vi "Page_Advanced_ReadAll.vi"(6 "ctl references":T1, 8 "error in (no error)":errorcluster, 10 "Calculated IncludeHWConfig":bool, 11 "AB_DLL in":refnum<class "AB_DLL.lvclass">) -> (0 "error out":errorcluster, 3 "AB_DLL out":refnum<class "AB_DLL.lvclass">)   [LabVIEW 2020, in "AB_DLL.lvclass"]
uses:
  <vilib>/AppBuilder/AB_Classes/DLL/AB_DLL.lvclass
  e:/builds/penguin/labview/branches/2020/dev/dist/vi.lib/AppBuilder/AB_Classes/TargetFile/AB_Targetfile.lvclass
  <resource>/Framework/Providers/Builds/AppBuilder/AB_UI_Page_Advanced_References.ctl
  <vilib>/AppBuilder/AB_Classes/DLL/AB_DLL.lvclass/AB_DLL.ctl
  <vilib>/AppBuilder/AB_Classes/Application/AB_Application.lvclass
  <vilib>/AppBuilder/AB_Classes/TargetFile/AB_Targetfile.lvclass
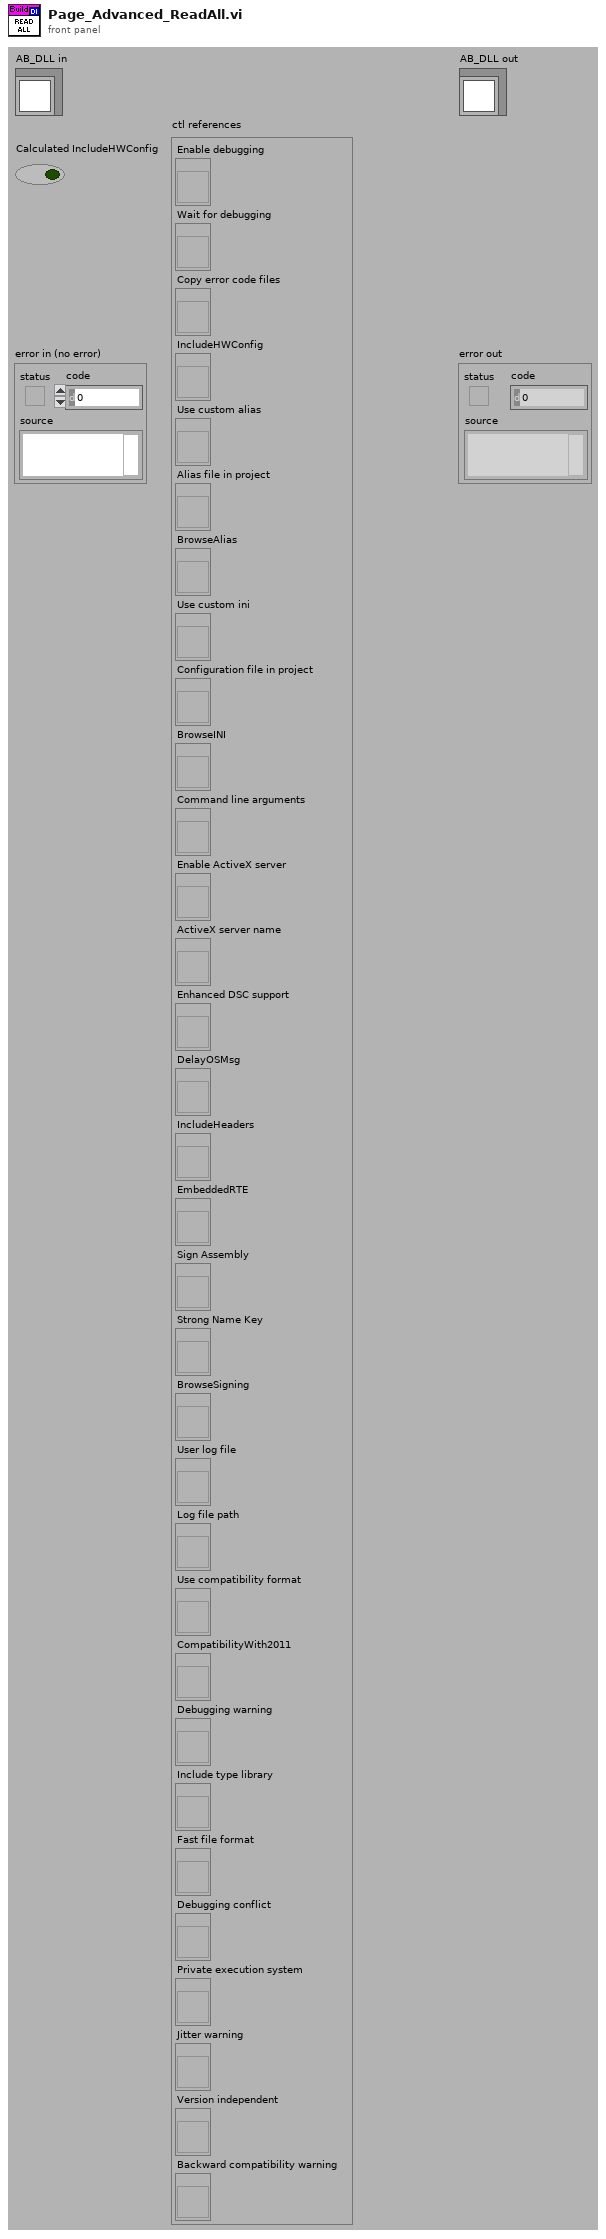
[diagram p1: front panel]
types:
  T1 = typedef "AB_UI_Page_Advanced_References.ctl" = cluster{"Enable debugging":refnum<vi>, "Wait for debugging":refnum<vi>, "Copy error code files":refnum<vi>, "IncludeHWConfig":refnum<vi>, "Use custom alias":refnum<vi>, "Alias file in project":refnum<vi>, "BrowseAlias":refnum<vi>, "Use custom ini":refnum<vi>, "Configuration file in project":refnum<vi>, "BrowseINI":refnum<vi>, "Command line arguments":refnum<vi>, "Enable ActiveX server":refnum<vi>, "ActiveX server name":refnum<vi>, "Enhanced DSC support":refnum<vi>, "DelayOSMsg":refnum<vi>, "IncludeHeaders":refnum<vi>, "EmbeddedRTE":refnum<vi>, "Sign Assembly":refnum<vi>, "Strong Name Key":refnum<vi>, "BrowseSigning":refnum<vi>, "User log file":refnum<vi>, "Log file path":refnum<vi>, "Use compatibility format":refnum<vi>, "CompatibilityWith2011":refnum<vi>, "Debugging warning":refnum<vi>, "Include type library":refnum<vi>, "Fast file format":refnum<vi>, "Debugging conflict":refnum<vi>, "Private execution system":refnum<vi>, "Jitter warning":refnum<vi>, "Version independent":refnum<vi>, "Backward compatibility warning":refnum<vi>}
  T2 = typedef "AB_Targetfile.ctl" = cluster{"targetfileName":string, "targetfileGUID":string, "enableDebugging":bool, "versionInfo":cluster{"productName":string, "legalCopyright":string, "companyName":string, "internalName":string, "fileDescription":string}, "eng_consolidatedTypeInfo":string, "fastFileFormat":bool, "eng_LEIFBuildData":u32, "versionIndependent":bool}
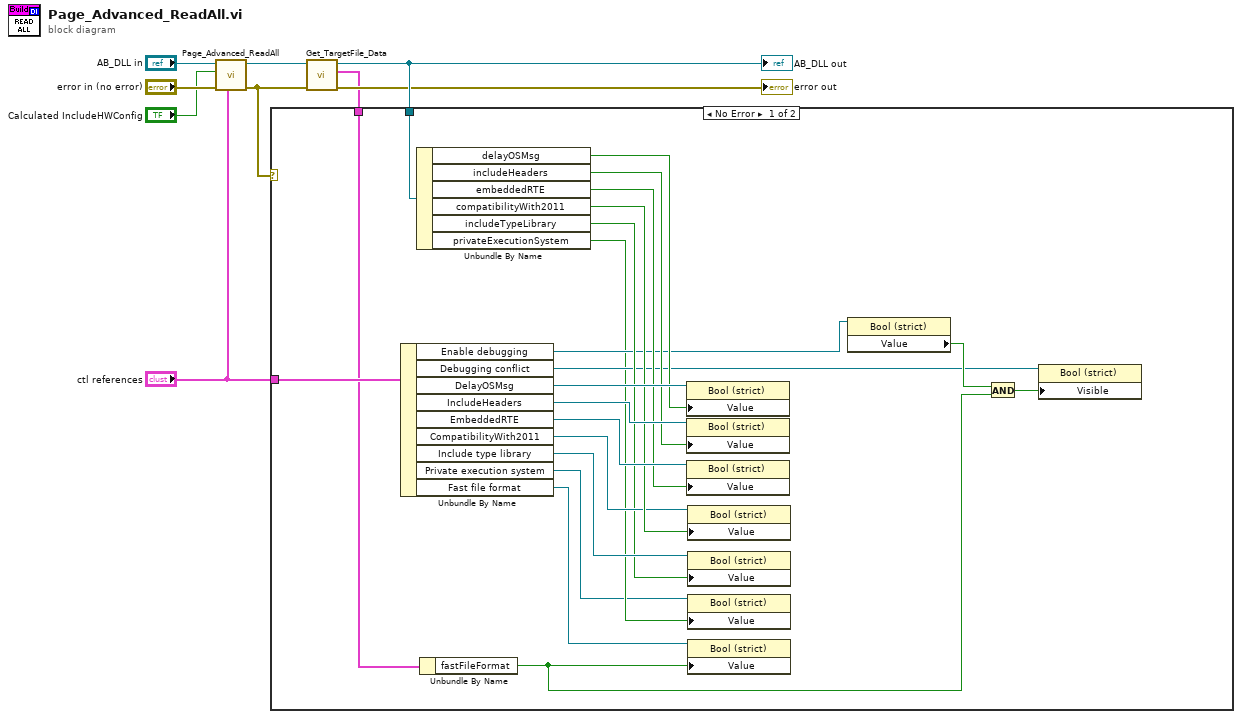
[diagram p0: block diagram]
diagram:
  n1 = call-parent "Page_Advanced_ReadAll.vi"("ctl references"="ctl references", "error in (no error)"="error in (no error)", "Calculated IncludeHWConfig"="Calculated IncludeHWConfig", "AB_Application in"="AB_DLL in") -> ("error out"=w3:errorcluster, "AB_Application out"=w5:refnum<class "AB_DLL.lvclass">)  [unwired: 6 in]
  n2 = call <vilib>:"Get_TargetFile_Data.vi"("error in (no error)"=w3, "AB_Targetfile in"=w5) -> ("error out"=→"error out":errorcluster, "data"=w1:T2, "AB_Targetfile out"=w4:refnum<class "AB_DLL.lvclass">)  [unwired: 7 in]
  "AB_DLL out" <- w4
  n3 = case shown="No Error" w3 {
    tunnel: w4 -> [w30 _]
    tunnel: "ctl references" -> [w29 _]
    tunnel: w1 -> [w18 _]
    frame No Error {
      n4 = Unbundle By Name(w29) -> ("Enable debugging"=w17:refnum<vi>, "Debugging conflict"=w15:refnum<vi>, "DelayOSMsg"=w28:refnum<vi>, "IncludeHeaders"=w26:refnum<vi>, "EmbeddedRTE"=w24:refnum<vi>, "CompatibilityWith2011"=w21:refnum<vi>, "Include type library"=w20:refnum<vi>, "Private execution system"=w11:refnum<vi>, "Fast file format"=w10:refnum<vi>)
      n5 = Unbundle By Name(w30) -> ("delayOSMsg"=w27:bool, "includeHeaders"=w25:bool, "embeddedRTE"=w23:bool, "compatibilityWith2011"=w22:bool, "includeTypeLibrary"=w19:bool, "privateExecutionSystem"=w12:bool)
      n6 = Unbundle By Name(w18) -> ("fastFileFormat"=w13:bool)
      n7 = property class="Bool (strict)"(reference=w28, "Value"=w27) -> ()  [unwired: 1 in, 2 out]
      n8 = property class="Bool (strict)"(reference=w26, "Value"=w25) -> ()  [unwired: 1 in, 2 out]
      n9 = property class="Bool (strict)"(reference=w24, "Value"=w23) -> ()  [unwired: 1 in, 2 out]
      n10 = property class="Bool (strict)"(reference=w21, "Value"=w22) -> ()  [unwired: 1 in, 2 out]
      n11 = property class="Bool (strict)"(reference=w20, "Value"=w19) -> ()  [unwired: 1 in, 2 out]
      n12 = property class="Bool (strict)"(reference=w11, "Value"=w12) -> ()  [unwired: 1 in, 2 out]
      n13 = property class="Bool (strict)"(reference=w10, "Value"=w13) -> ()  [unwired: 1 in, 2 out]
      n14 = property class="Bool (strict)"(reference=w17) -> ("Value"=w16:bool)  [unwired: 1 in, 2 out]
      n15 = And(x=w16, y=w13) -> (x .and. y?=w14:bool)
      n16 = property class="Bool (strict)"(reference=w15, "Visible"=w14) -> ()  [unwired: 1 in, 2 out]
    }
    frame Error {
    }
  }
